vi "openDevice.vi"(8 "error in (no error)":errorcluster, 10 "deviceName":string, 11 "BECHWCBasic in":refnum<class "BECHWCBasic.lvclass">) -> (0 "error out":errorcluster, 3 "BECHWCBasic out":refnum<class "BECHWCBasic.lvclass">)   [LabVIEW 2011, in "Hardware.lvlib" / "HWControllers.lvlib" / "BECHWCBasic.lvclass"]
doc: "Opens a device."
uses:
  BECHWCBasic.lvclass
  IntegrationManagement/CameraManager.lvclass
  BECHWCBasic.lvclass/BECHWCBasic.ctl
  HWController.lvclass
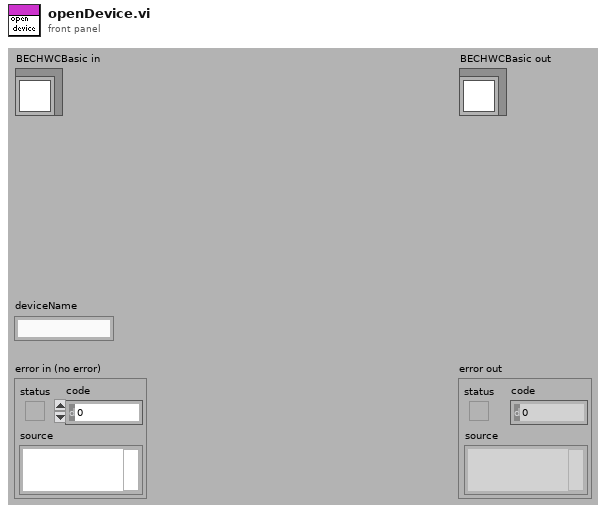
[diagram p1: front panel]
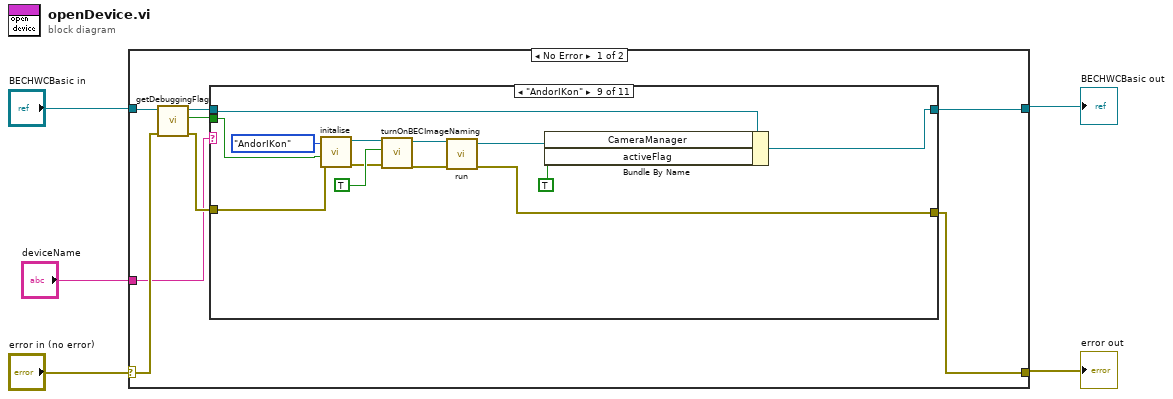
[diagram p0: block diagram]
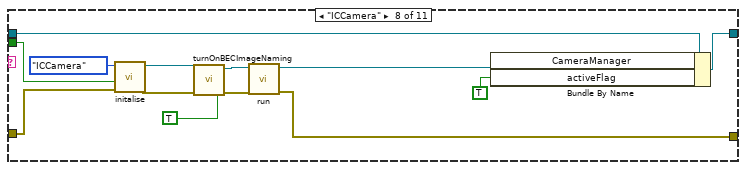
[diagram p9: hidden frame]
diagram:
  n1 = case shown="No Error" "error in (no error)" {
    selector: "error in (no error)" -> [w9 w59]
    tunnel: [w6 w59] -> w4
    tunnel: [w7 w58] -> w2
    tunnel: "BECHWCBasic in" -> [w13 w58]
    tunnel: "deviceName" -> [w8 _]
    frame No Error {
      n2 = call "getDebuggingFlag.vi"("error in (no error)"=w9, "HWController.lvclass in"=w13) -> ("error out"=w10:errorcluster, "debuggingFlag"=w11:bool, "HWController.lvclass out"=w12:refnum<class "BECHWCBasic.lvclass">)  [unwired: 7 in]
      n3 = case shown="\"AndorIKon\"" w8 {
        tunnel: w12 -> [w15 w17 w19 w21 w22 w25 w27 w38 w51 w55 w57]
        tunnel: [w15 w17 w19 w21 w22 w25 w27 w39 w52 w55 w57] -> w7
        tunnel: w10 -> [w14 w16 w18 w20 w23 w24 w26 w36 w50 w54 w56]
        tunnel: [w14 w16 w18 w20 w23 w24 w26 w33 w48 w54 w56] -> w6
        tunnel: w11 -> [_ _ _ _ _ _ _ w37 w41 _ _]
        frame "No Hardware", Default {
        }
        frame "UsbDAQ" {
        }
        frame "Daq" {
        }
        frame "Dio64" {
        }
        frame "Ao8" {
        }
        frame "Ao32" {
        }
        frame "ArbWave" {
        }
        frame "ICCamera" {
          n4 = call "initalise.vi"("error in (no error)"=w36, "Hardware Connected?"=w37, "Camera"=enum16{"AndorIKon", "ICCamera"}."ICCamera") -> ("error out"=w32:errorcluster, "CameraManager out"=w31:refnum<class "CameraManager.lvclass">)  [unwired: 7 in]
          n5 = call "turnOnBECImageNaming.vi"("error in (no error)"=w32, "ImageRenaming"=TRUE, "CameraManager in"=w31) -> ("error out"=w29:errorcluster, "CameraManager out"=w30:refnum<class "CameraManager.lvclass">)  [unwired: 7 in]
          n6 = call-dynamic "run.vi"("error in (no error)"=w29, "CameraManager in"=w30) -> ("error out"=w33:errorcluster, "CameraManager out"=w34:refnum<class "CameraManager.lvclass">)  [unwired: 8 in]
          n7 = Bundle By Name(cluster=w38, "CameraManager"=w34, "activeFlag"=TRUE) -> (w39:refnum<class "BECHWCBasic.lvclass">)
        }
        frame "AndorIKon" {
          n8 = call "initalise.vi"("error in (no error)"=w50, "Hardware Connected?"=w41, "Camera"=enum16{"AndorIKon", "ICCamera"}."AndorIKon") -> ("error out"=w45:errorcluster, "CameraManager out"=w44:refnum<class "CameraManager.lvclass">)  [unwired: 7 in]
          n9 = call "turnOnBECImageNaming.vi"("error in (no error)"=w45, "ImageRenaming"=TRUE, "CameraManager in"=w44) -> ("error out"=w42:errorcluster, "CameraManager out"=w43:refnum<class "CameraManager.lvclass">)  [unwired: 7 in]
          n10 = call-dynamic "run.vi"("error in (no error)"=w42, "CameraManager in"=w43) -> ("error out"=w48:errorcluster, "CameraManager out"=w49:refnum<class "CameraManager.lvclass">)  [unwired: 8 in]
          n11 = Bundle By Name(cluster=w51, "CameraManager"=w49, "activeFlag"=TRUE) -> (w52:refnum<class "BECHWCBasic.lvclass">)
        }
        frame "S1010" {
        }
        frame "C100" {
        }
      }
    }
    frame Error {
    }
  }
  "error out" <- w4
  "BECHWCBasic out" <- w2
